vi "StageStopMove.vi"(8 "error in (no error)":errorcluster, 10 "Stage events":refnum<queue>, 11 "Microscope in":refnum<class "Microscope.lvclass">) -> (0 "error out":errorcluster, 3 "Microscope out":refnum<class "Microscope.lvclass">)   [LabVIEW 2012, in "Microscope.lvclass"]
uses:
  classes/Microscope.lvclass
  typedefs/StageEvent.ctl
  typedefs/Move Type.ctl
  classes/Microscope.lvclass/Microscope.ctl
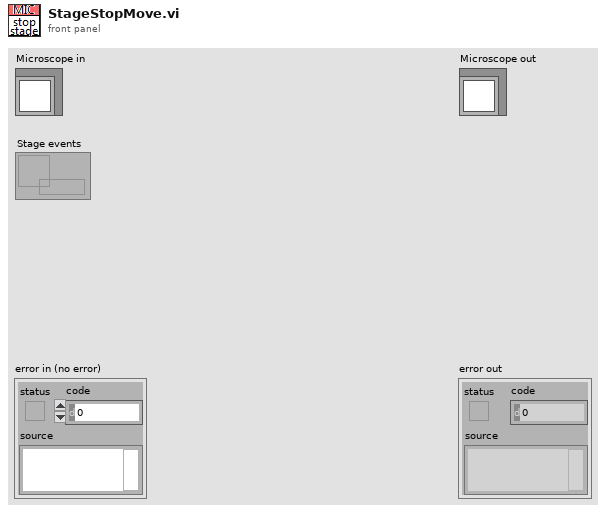
[diagram p1: front panel]
types:
  T1 = typedef "Move Type.ctl" = enum16{"None", "Continuous", "Discrete"}
  T2 = typedef "StageEvent.ctl" = enum16{"stage.TimeOut", "stage.FlushData", "stage.GetPosition", "stage.Init", "stage.MoveTo1", "stage.MoveTo2", "stage.MoveTo3", "stage.Stop"}
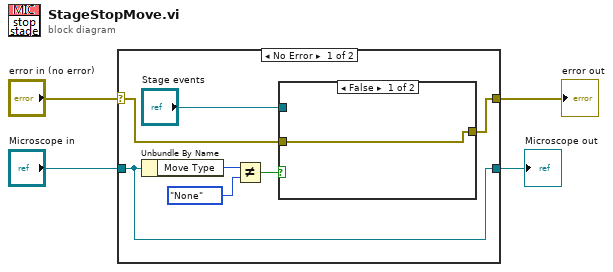
[diagram p0: block diagram]
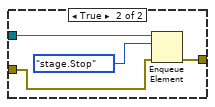
[diagram p2: hidden frame]
diagram:
  n1 = case shown="No Error" "error in (no error)" {
    selector: "error in (no error)" -> [w6 w18]
    tunnel: [w5 w18] -> w3
    tunnel: [w11 w17] -> w1
    tunnel: "Microscope in" -> [w11 w17]
    frame No Error {
      n2 = Unbundle By Name(w11) -> ("Move Type"=w10:T1)
      n3 = Not Equal?(x=w10, y=Move_Type."None") -> (x != y?=w9:bool)
      n4 = case shown="False" w9 {
        tunnel: "Stage events" -> [_ w16]
        tunnel: w6 -> [w12 w14]
        tunnel: [w12 w13] -> w5
        frame False {
        }
        frame True {
          n5 = Enqueue Element(queue=w16, element=StageEvent."stage.Stop", error in (no error)=w14) -> (error out=w13:errorcluster)  [unwired: 1 in, 2 out]
        }
      }
    }
    frame Error {
    }
  }
  "error out" <- w3
  "Microscope out" <- w1
